vi "IMAQToPythonImage.vi"(8 "error in (no error)":errorcluster, 11 "IMAQ Image in":T1) -> (0 "error out":errorcluster, 2 "Python Image Data":u8[][][](array[numeric]), 3 "IMAQ Image dup":T1)   [LabVIEW 2017, in "ImageFacialDetection.lvclass"]
doc: "Converts a LabVIEW 2D picture to a Python image - a 3D array with\ndimensions (height, width, color)."
uses:
  ImageFacialDetection.lvclass
  <vilib>/vision/Image Controls.llb/IMAQ Image.ctl
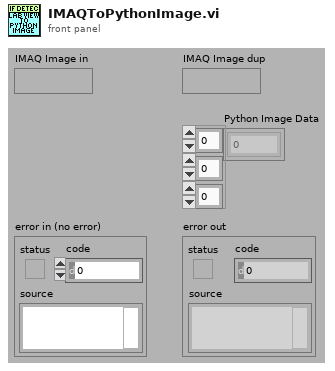
[diagram p1: front panel]
types:
  T1 = typedef "IMAQ Image.ctl" = refnum<image>
  T2 = typedef "imagedata.ctl" = cluster{"image type":i32, "image depth":i32, "image":u8[], "mask":u8[], "colors":u32[], "Rectangle":cluster{"left":i16, "top":i16, "right":i16, "bottom":i16}}
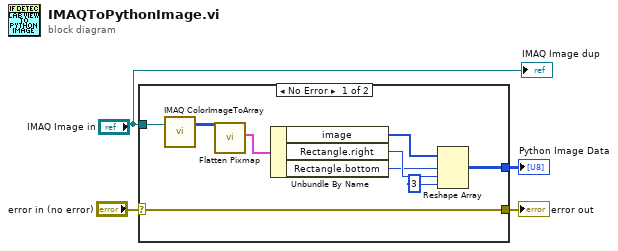
[diagram p0: block diagram]
diagram:
  n1 = case shown="No Error" "error in (no error)" {
    selector: "error in (no error)" -> [w13 w14]
    tunnel: [w13 w14] -> w3
    tunnel: "IMAQ Image in" -> [w5 _]
    tunnel: [w8 _] -> w2
    frame No Error {
      n2 = call "IMAQ ColorImageToArray"("Image"=w5) -> ("Image Pixels (U32)"=w7:u32[][])  [unwired: 3 in, 2 out]
      n3 = call <vilib>:"Flatten Pixmap.vi"("24-bit pixmap"=w7) -> ("image data"=w6:T2)  [unwired: 10 in]
      n4 = Unbundle By Name(w6) -> ("image"=w12:u8[], "Rectangle.right"=w10:i16, "Rectangle.bottom"=w9:i16)
      n5 = Reshape Array(w12, w9, w10, 3 ("dimension size")) -> (w8:u8[][][])
    }
    frame Error {
    }
  }
  "error out" <- w3
  "Python Image Data" <- w2
  "IMAQ Image dup" <- "IMAQ Image in"
